vi "check_signal_chopper_state.vi"(7 "parity?":bool, 10 "chopper signal":bool[](array[boolean]), 11 "data_raw_signal":dbl[][](array[numeric])) -> (2 "chopper signal 2":bool[](array[boolean]), 3 "data_raw_signal 2":dbl[][](array[numeric]))   [LabVIEW 2019]
panel:
  out "chopper reference 2":bool[](array[boolean])
  out "data_raw_reference 2":dbl[][](array[numeric])
  in  "chopper reference":bool[](array[boolean])
  in  "data_raw_reference":dbl[][](array[numeric])
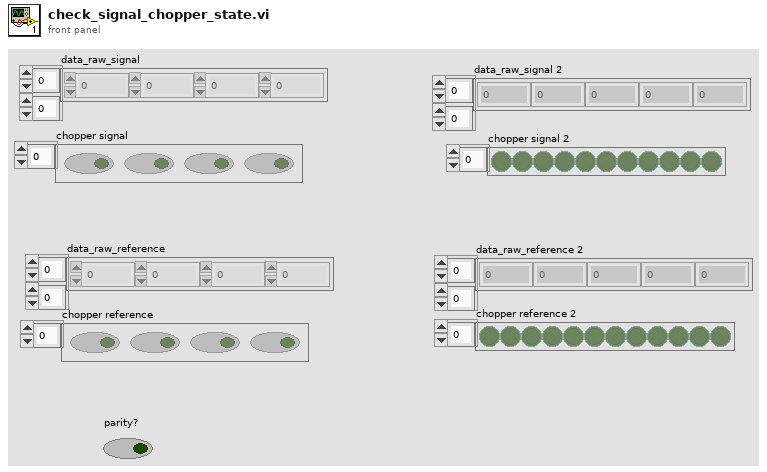
[diagram p1: front panel]
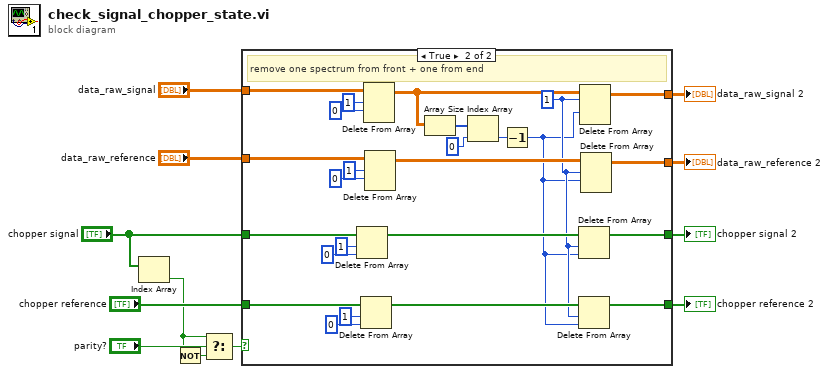
[diagram p0: block diagram]
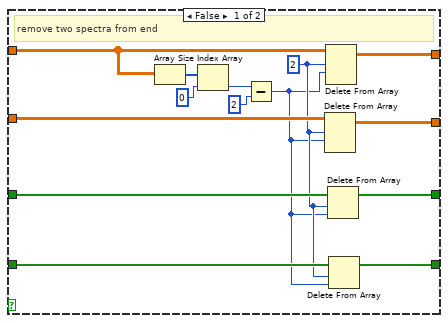
[diagram p2: hidden frame]
diagram:
  n1 = Index Array(array="chopper signal") -> (element=w2:bool)  [unwired: 1 in]
  n2 = Not(x=w2) -> (.not. x?=w1:bool)
  n3 = Select(t=w2, s="parity?", f=w1) -> (s? t:f=w4:bool)
  n4 = case shown="True" w4 {
    tunnel: "data_raw_signal" -> [w21 w40]
    tunnel: "data_raw_reference" -> [w23 w51]
    tunnel: [w22 w44] -> w8
    tunnel: [w24 w46] -> w9
    tunnel: "chopper signal" -> [w18 w34]
    tunnel: "chopper reference" -> [w17 w33]
    tunnel: [w14 w28] -> w7
    tunnel: [w13 w27] -> w6
    frame False {
      w16 = 2 ("length")
      # "remove two spectra from end"
      n5 = Array Size(array=w21) -> (size(s)=w26:i32[])
      n6 = Index Array(array=w26, index=0) -> (element=w20:i32)
      n7 = Subtract(x=w20, y=2) -> (x-y=w15:i32)
      n8 = Delete From Array(array=w23, length=w16, index (row)=w15) -> (array with subset deleted=w22:dbl[][])  [unwired: 1 in, 1 out]
      n9 = Delete From Array(array=w21, length=w16, index (row)=w15) -> (array with subset deleted=w24:dbl[][])  [unwired: 1 in, 1 out]
      n10 = Delete From Array(array=w18, length=w16, index=w15) -> (array with subset deleted=w14:bool[])  [unwired: 1 out]
      n11 = Delete From Array(array=w17, length=w16, index=w15) -> (array with subset deleted=w13:bool[])  [unwired: 1 out]
    }
    frame True {
      w30 = 1 ("length")
      # "remove one spectrum from front + one from end"
      n12 = Delete From Array(array=w34, length=1, index=0 ("index (row)")) -> (array with subset deleted=w32:bool[])  [unwired: 1 out]
      n13 = Delete From Array(array=w33, length=1, index=0 ("index (row)")) -> (array with subset deleted=w31:bool[])  [unwired: 1 out]
      n14 = Delete From Array(array=w40, length=1, index (row)=0) -> (array with subset deleted=w39:dbl[][])  [unwired: 1 in, 1 out]
      n15 = Delete From Array(array=w51, length=1, index (row)=0) -> (array with subset deleted=w45:dbl[][])  [unwired: 1 in, 1 out]
      n16 = Array Size(array=w39) -> (size(s)=w43:i32[])
      n17 = Index Array(array=w43, index=0) -> (element=w41:i32)
      n18 = Decrement(x=w41) -> (x-1=w29:i32)
      n19 = Delete From Array(array=w32, length=w30, index=w29) -> (array with subset deleted=w28:bool[])  [unwired: 1 out]
      n20 = Delete From Array(array=w31, length=w30, index=w29) -> (array with subset deleted=w27:bool[])  [unwired: 1 out]
      n21 = Delete From Array(array=w39, length=w30, index (row)=w29) -> (array with subset deleted=w46:dbl[][])  [unwired: 1 in, 1 out]
      n22 = Delete From Array(array=w45, length=w30, index (row)=w29) -> (array with subset deleted=w44:dbl[][])  [unwired: 1 in, 1 out]
    }
  }
  "data_raw_signal 2" <- w9
  "data_raw_reference 2" <- w8
  "chopper signal 2" <- w7
  "chopper reference 2" <- w6
